vi "FFT.vi"(8 "error in (no error)":errorcluster, 9 "SubQueueIN":refnum<queue>, 10 "MainQueueIN":refnum<queue>, 11 "Data Value Reference IN":refnum<data-value>) -> (0 "error out":errorcluster, 3 "Data Value Reference out":refnum<data-value>)   [LabVIEW 2013]
uses:
  Control/SystemCommand.ctl
  Control/SystemData.ctl
  Control/SignalType.ctl
  Control/SubDaqCommand.ctl
  <vilib>/Analysis/4window.llb/windowTd.ctl
  <vilib>/measure/maspectr.llb/FFT Spectrum (Mag-Phase) for N Chan.vi
  <vilib>/measure/NI_MAPro.lvlib
  <vilib>/Analysis/NI_AALPro.lvlib
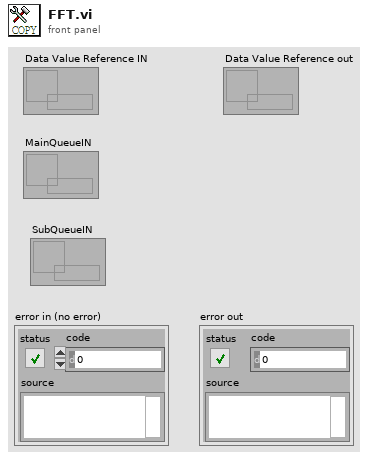
[diagram p1: front panel]
types:
  T1 = cluster{"averaging mode":enum16{"No averaging", "Vector averaging", "RMS averaging", "Peak hold"}, "weighting mode":enum16{"Linear", "Exponential"}, "number of averages":u32}
  T2 = cluster{"dB On (F)":bool, "unwrap phase (F)":bool, "convert to degree (F)":bool}
  T3 = typedef "NI_AALPro.lvlib/windowTd.ctl" = u32
  T4 = typedef "SystemData.ctl" = cluster{"Numeric":dbl, "String":string, "Boolean":bool, "Frequency":dbl, "Amplitude":dbl, "SignalType":T5, "WaveformArray":waveform(dbl)[], "Reset":bool, "StateString":string, "FFTmagnitudes":cluster{"f0":dbl, "df":dbl, "magnitude":dbl[]}[]}
  T5 = typedef "SignalType.ctl" = enum16{"Sin", "Triangle", "Square"}
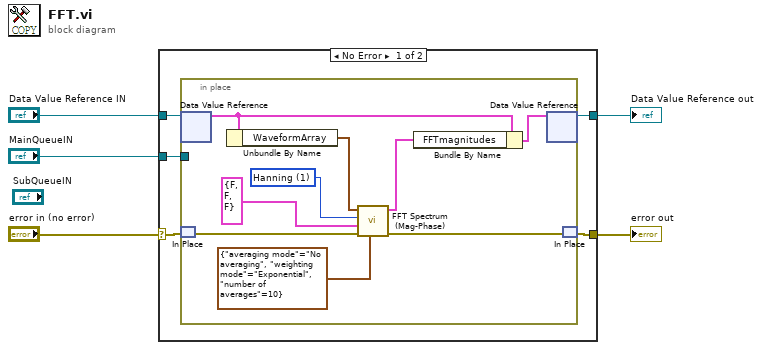
[diagram p0: block diagram]
diagram:
  n1 = case shown="No Error" "error in (no error)" {
    selector: "error in (no error)" -> [w8 w20]
    tunnel: "Data Value Reference IN" -> [w10 w21]
    tunnel: [w9 w21] -> w2
    tunnel: [w7 w20] -> w4
    tunnel: "MainQueueIN" -> [w6 _]
    frame No Error {
      n2 = in-place {
        in-place-border: w6 -> [_]
        w17 = T3 1 items=["Rectangle"=0, "Hanning"=1, "Hamming"=2, "Blackman-Harris"=3, "Exact Blackman"=4, "Blackman"=5, "Flat Top"=6, "4 Term B-Harris "=7, "7 Term B-Harris"=8, "Low Sidelobe"=9, "Blackman Nuttall"=11, "Triangle"=30, "Bartlett-Hanning"=31, "Bohman"=32, "Parzen"=33, "Welch"=34, "Kaiser"=60, "Dolph-Chebyshev"=61, "Gaussian"=62] ("window")
        n3 = in-place-dvr #1(w10) -> (w13:T4)  [unwired: 1 out]
        n4 = in-place-match #2(w8) -> (w19:errorcluster)
        n5 = Unbundle By Name(w13) -> ("WaveformArray"=w18:waveform(dbl)[])
        n6 = call-poly <vilib>:"FFT Spectrum (Mag-Phase).vi"("averaging parameters"=T1 {"averaging mode"=enum."No averaging", "weighting mode"=enum."Exponential", "number of averages"=10}, "error in (no error)"=w19, "view"=T2 {"dB On (F)"=FALSE, "unwrap phase (F)"=FALSE, "convert to degree (F)"=FALSE}, "window"=w17, "time signals"=w18) -> ("error out"=w14:errorcluster, "magnitudes"=w11:cluster{"f0":dbl, "df":dbl, "magnitude":dbl[]}[])  [unwired: 2 in, 3 out]
        n7 = Bundle By Name(cluster=w13, "FFTmagnitudes"=w11) -> (w12:T4)
        n8 = in-place-dvr #1(w12) -> (w9:refnum<data-value>)  [unwired: 1 out]
        n9 = in-place-match #2(w14) -> (w7:errorcluster)
      }
    }
    frame Error {
    }
  }
  "error out" <- w4
  "Data Value Reference out" <- w2
